vi "which_drug_port.vi"(7 "DILUTION COLUMN":dbl[](array[numeric]), 10 "1X PORT":i32, 11 "17X PORT":i32) -> (3 "DRUG PORT":i32)   [LabVIEW 2013]
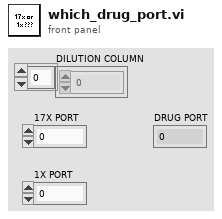
[diagram p1: front panel]
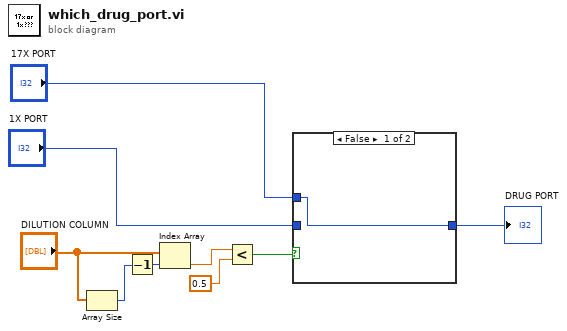
[diagram p0: block diagram]
diagram:
  n1 = Array Size(array="DILUTION COLUMN") -> (size(s)=w5:i32)
  n2 = Decrement(x=w5) -> (x-1=w4:i32)
  n3 = Index Array(array="DILUTION COLUMN", index=w4) -> (element=w2:dbl)
  n4 = Less?(x=w2, y=0.5) -> (x < y?=w1:bool)
  n5 = case shown="False" w1 {
    tunnel: "17X PORT" -> [w10 _]
    tunnel: [w10 w11] -> w9
    tunnel: "1X PORT" -> [_ w11]
    frame False {
    }
    frame True {
    }
  }
  "DRUG PORT" <- w9
